vi "Close.vi"(8 "error in (no error)":errorcluster, 9 "Stop Event":refnum<user-event>, 10 "Sequence Context":refnum<k7>, 11 "TestExec in":refnum<class "TestExec.lvclass">) -> (0 "error out":errorcluster, 3 "TestExec out":refnum<class "TestExec.lvclass">)   [LabVIEW 2019, in "OPC UA.lvlib" / "TestExec.lvclass"]
uses:
  TestExec.lvclass
  TestExec.lvclass/TestExec.ctl
  OPC UA/OPC UA.lvclass
  <vilib>/addons/TestStand/_TSUtility.llb/TestStand - Set Property Value (Boolean).vi
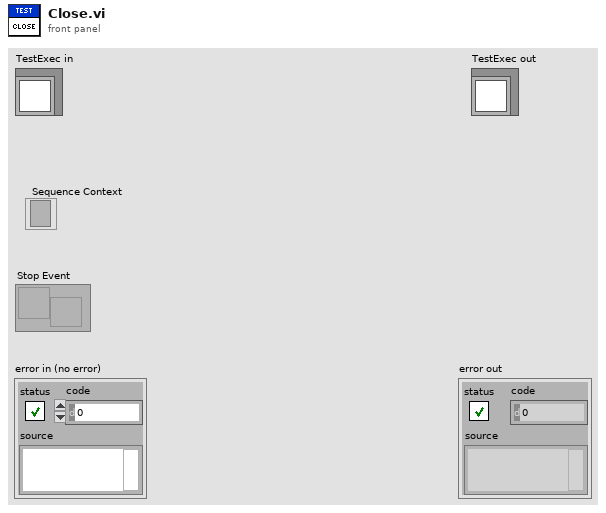
[diagram p1: front panel]
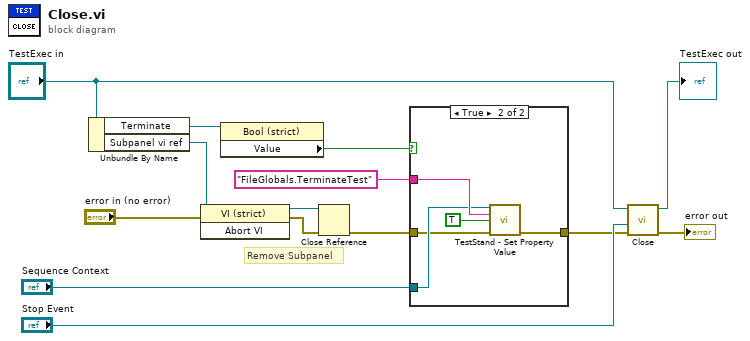
[diagram p0: block diagram]
diagram:
  # "Remove Subpanel"
  n1 = Unbundle By Name("TestExec in") -> ("Terminate"=w6:refnum<vi>, "Subpanel vi ref"=w9:refnum<vi>)
  n2 = invoke on="Invoke Node" class="VI (strict)" method="Abort VI"(reference=w9, error in="error in (no error)") -> (reference out=w10:refnum<vi>, error out=w12:errorcluster)  [unwired: 1 in, 1 out]
  n3 = property class="Bool (strict)"(reference=w6) -> ("Value"=w5:bool)  [unwired: 1 in, 2 out]
  n4 = Close Reference(reference=w10, error in (no error)=w12) -> (error out=w2:errorcluster)
  n5 = case shown="True" w5 {
    tunnel: "FileGlobals.TerminateTest" ("Lookup String") -> [_ w19]
    tunnel: "Sequence Context" -> [_ w18]
    tunnel: w2 -> [w15 w17]
    tunnel: [w15 w16] -> w1
    frame False {
    }
    frame True {
      n6 = call-poly <vilib>:"TestStand - Set Property Value.vi"("Sequence Context In"=w18, "Lookup String"=w19, "New Value"=TRUE, "error in (no error)"=w17) -> ("error out"=w16:errorcluster)  [unwired: 10 in, 1 out]
    }
  }
  n7 = call-parent "Close.vi"("error in (no error)"=w1, "Stop Event"="Stop Event", "OPC UA in"="TestExec in") -> ("error out"=→"error out":errorcluster, "OPC UA out"=→"TestExec out":refnum<class "TestExec.lvclass">)  [unwired: 7 in]
